vi "RSNRPZ Error Message.vi"(8 "error in (no error)":errorcluster, 10 "Status Code (0)":i32, 11 "VISA session":refnum<visa-resource-name> caption="VISA resource name") -> (0 "error out":errorcluster, 2 "Message":string, 3 "dup VISA session":refnum<visa-resource-name> caption="VISA resource name")   [LabVIEW 2010]
doc: "This VI takes the Status Code returned by the instrument driver VIs, interprets it and returns it as a user readable string."
uses:
  rsnrpz_32.dll
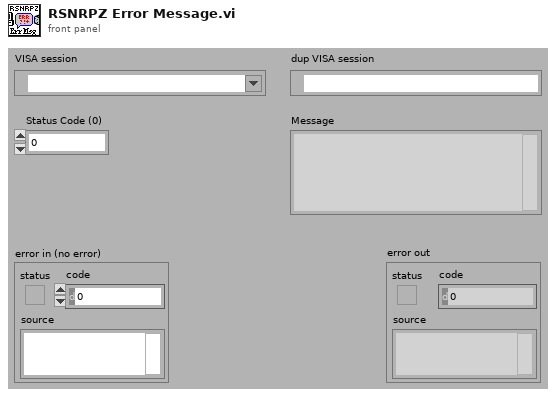
[diagram p1: front panel]
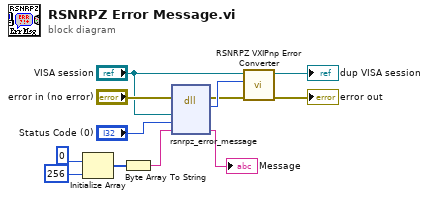
[diagram p0: block diagram]
diagram:
  n1 = Initialize Array(u8 0, 256) -> (w10:u8[])
  n2 = Byte Array To String(unsigned byte array=w10) -> (string=w7:string)
  n3 = dll-call lib="rsnrpz_32.dll" fn="rsnrpz_error_message"(error in="error in (no error)", "VISA Session"="VISA session", "Status Code"="Status Code (0)", "Message"=w7) -> (error out=w5:errorcluster, "Status"=w9:i32, "Message"=→"Message":string)  [unwired: 4 in, 1 out]
  n4 = call <instrlib>:"RSNRPZ VXIPnp Error Converter.vi"("error in"=w5, "VXIPnp error code"=w9, "VISA session"="VISA session") -> ("error out"=→"error out":errorcluster, "dup VISA session"=→"dup VISA session":refnum<visa-resource-name>)  [unwired: 7 in]
